vi "Config AI.vi"(6 "Channel config":T1={"Channel"="", "Vmax"=5.0, "Vmin"=-5.0, "name to assign"="", "input terminal configuration"=10083} {"input terminal configuration" items=["Default"=-1, "RSE"=10083, "NRSE"=10078, "Differential"=10106, "Pseudodifferential"=12529]; "Vmin" format="%0.2f"; "Vmax" format="%0.2f"}, 8 "error in":errorcluster, 11 "task in":refnum<k21>) -> (0 "error out":errorcluster, 3 "task out":refnum<k21>)   [LabVIEW 2019]
doc: "This example demonstrates how to acquire a continuous amount of data (Waveform) using the DAQ device's internal clock. It also shows how to synchronize two devices for different device families (E Series, S Series, M Series, X Series, DSA, and SC Express), to simultaneously acquire the data.\n\nFor instructions on how to connect your signals to the DAQ device, refer to your device documentation."
uses:
  <vilib>/DAQmx/create/channels.llb/DAQmx Create Channel (AI-Voltage-Basic).vi
panel:
  # "Config AI"
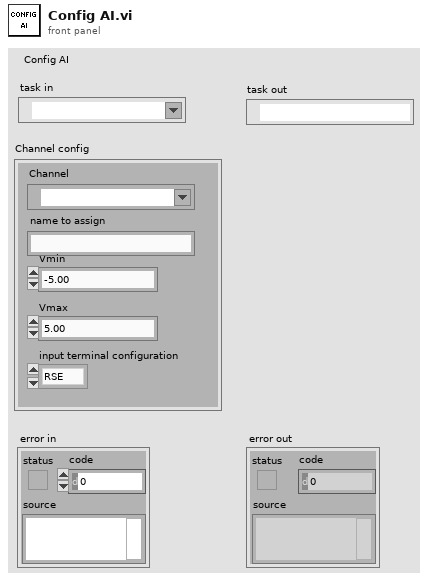
[diagram p1: front panel]
types:
  T1 = cluster{"Channel":tag, "Vmax":dbl, "Vmin":dbl, "name to assign":string, "input terminal configuration":i32}
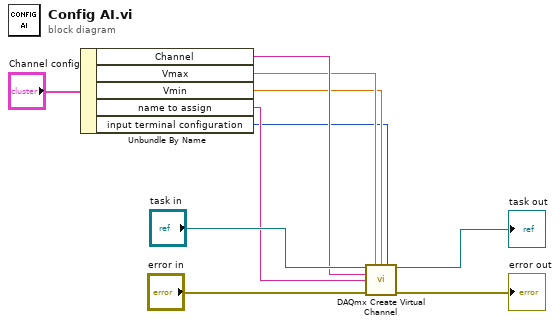
[diagram p0: block diagram]
diagram:
  n1 = Unbundle By Name("Channel config") -> ("Channel"=w5:tag, "Vmax"=w4:dbl, "Vmin"=w3:dbl, "name to assign"=w2:string, "input terminal configuration"=w1:i32)
  n2 = call-poly <vilib>:"DAQmx Create Virtual Channel.vi"("task in"="task in", "maximum value"=w4, "minimum value"=w3, "input terminal configuration"=w1, "physical channels"=w5, "name to assign"=w2, "error in"="error in") -> ("task out"=→"task out":refnum<k21>, "error out"=→"error out":errorcluster)  [unwired: 7 in]
